vi "TempSetpointSetup.vi"(0 "Elevator Switch":bool=TRUE, 2 "Enable Auto":bool=TRUE, 3 "Elevator Manual Power":dbl format="%#_13g", 4 "Wrist Manual Power":dbl format="%#_13g", 5 "Horse Drive Manual Power":dbl format="%#_13g", 6 "Elevator Level Select":T1(ring), 7 "Wrist":T4(ring), 8 "Cluster":T2={"Elevator Setpoints"=[], "Wrist Setpoints"=[], "Horse Drive Setpoints"=[], "Wrist Gains"={"proportional gain (Kc)"=1.0, "integral time (Ti, min)"=0.01, "derivative time (Td, min)"=0.0}, "Wrist Power Limits"={"output high"=0.25, "output low"=-0.25}, "Horse Gains"={"proportional gain (Kc)"=1.0, "integral time (Ti, min)"=0.01, "derivative time (Td, min)"=0.0}, "Horse Power Limits"={"output high"=0.25, "output low"=-0.25}, "Elevator Gains"={"proportional gain (Kc)"=1.0, "integral time (Ti, min)"=0.01, "derivative time (Td, min)"=0.0}, "Elevator Power Limits"={"output high"=0.25, "output low"=-0.25}}, 9 "Horse Drive":T3(ring)) -> (20 "Elevator Power Out":dbl, 21 "Wrist Power Out":dbl, 22 "Horse Drive Power Out":dbl)   [LabVIEW 2018]
uses:
  <vilib>/Rock Robotics/WPI/ThirdParty/Phoenix-LabVIEW/Motor Controller/Get/CTRE_Phoenix_MotorController_GetSelectedSensorData.vi
  Toolbox/Simple Limit Switch/Limits(SingleSwitch).vi
  Toolbox/Simple Limit Switch/Limits(DoubleSwitch).vi
  Toolbox/Simple Limit Switch/Limits(Switch+Encoder).vi
panel:
  out "Outer Lift Limit":i32
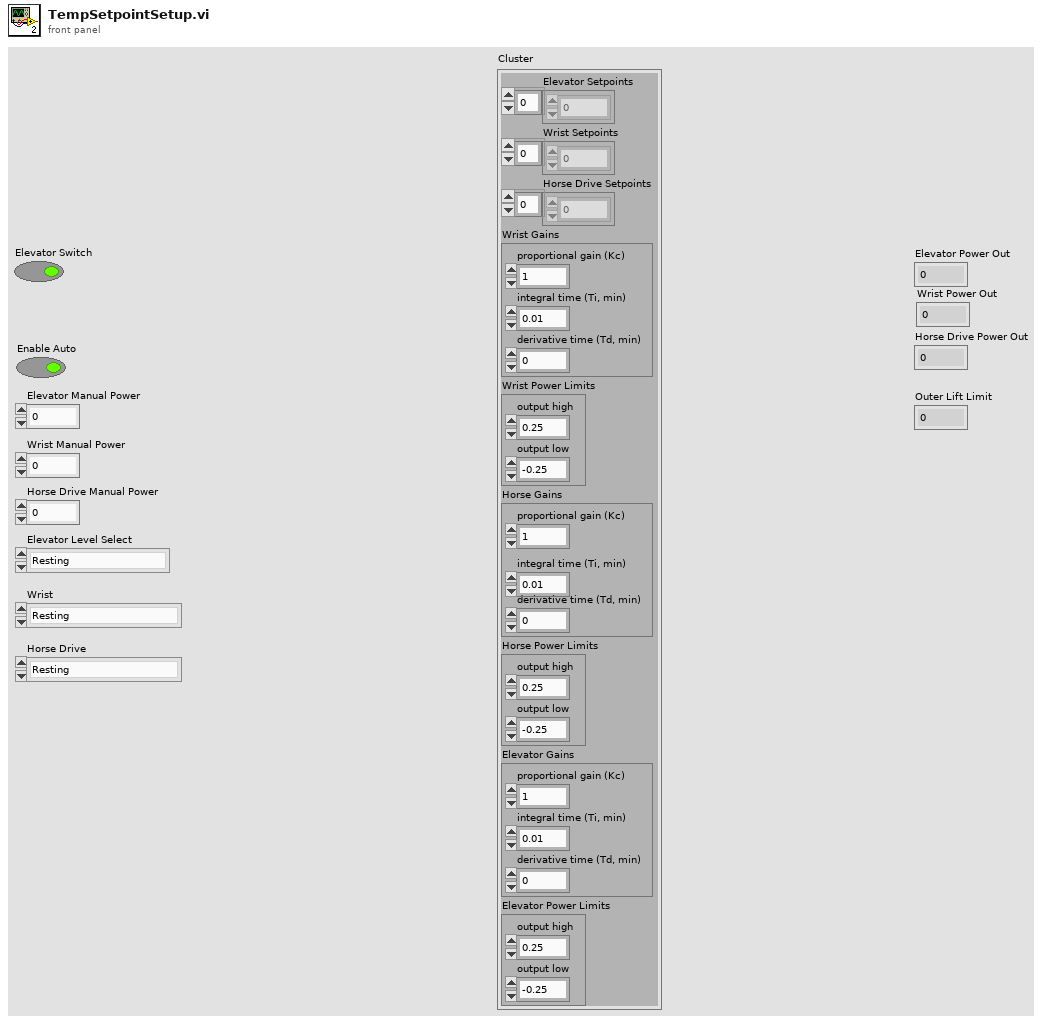
[diagram p1: front panel]
types:
  T1 = enum16{"Resting", "CargoShip Front", "CargoShip Back", "Cargo Mid", "Hatch Mid", "All High", "Cargo Intake"}
  T2 = cluster{"Elevator Setpoints":dbl[], "Wrist Setpoints":dbl[], "Horse Drive Setpoints":dbl[], "Wrist Gains":cluster{"proportional gain (Kc)":dbl, "integral time (Ti, min)":dbl, "derivative time (Td, min)":dbl}, "Wrist Power Limits":cluster{"output high":dbl, "output low":dbl}, "Horse Gains":cluster{"proportional gain (Kc)":dbl, "integral time (Ti, min)":dbl, "derivative time (Td, min)":dbl}, "Horse Power Limits":cluster{"output high":dbl, "output low":dbl}, "Elevator Gains":cluster{"proportional gain (Kc)":dbl, "integral time (Ti, min)":dbl, "derivative time (Td, min)":dbl}, "Elevator Power Limits":cluster{"output high":dbl, "output low":dbl}}
  T3 = enum16{"Resting", "PLACEHOLDER", "Hatch Intake", "Lift"}
  T4 = enum16{"Resting", "Hatch Ground Intake", "Hatch Place Low/Mid/CargoShip", "Hatch Place High", "Cargo Ground Intake", "Cargo Place Low/Mid", "Cargo Place High", "CargoShip Place Front", "CargoShip Place Back"}
  T5 = cluster{"proportional gain (Kc)":dbl, "integral time (Ti, min)":dbl, "derivative time (Td, min)":dbl}
  T6 = typedef "WPI_SwitchDevRef.ctl" = cluster{"DevStatus":errorcluster, "DIO Channel":T7, "CntIndex":T8, "Normally Closed":bool}
  T7 = typedef "FPGA_DIOChannel.ctl" = enum8{"DIO 0", "DIO 1", "DIO 2", "DIO 3", "DIO 4", "DIO 5", "DIO 6", "DIO 7", "DIO 8", "DIO 9", "DIO MXP 0", "DIO MXP 1", "DIO MXP 2", "DIO MXP 3", "DIO MXP 4", "DIO MXP 5", "DIO MXP 6", "DIO MXP 7", "DIO MXP 8", "DIO MXP 9", "DIO MXP 10", "DIO MXP 11", "DIO MXP 12", "DIO MXP 13", "DIO MXP 14", "DIO MXP 15", "SPI Port CS1", "SPI Port CS2", "SPI Port CS3", "SPI Port MISO", "SPI Port MOSI", "Invalid"}
  T8 = typedef "FPGA_CounterCtrSystemIndex.ctl" = enum8{"Ctr 0", "Ctr 1", "Ctr 2", "Ctr 3", "Ctr 4", "Ctr 5", "Ctr 6", "Ctr 7", "Invalid"}
  T9 = typedef "WPI_MotorControlDeviceRef.ctl" = cluster{"DeviceStatus":errorcluster, "Type":T10, "PWM":cluster{"PWM Channel":T11, "DeadBand":T12}, "CAN":cluster{"Device Number":u8, "SetOutput VI Ref":variant, "GetOutput VI Ref":variant, "Enable VI Ref":variant, "Disable VI Ref":variant, "Data":variant}, "Invert":bool, "DIO PWM":cluster{"PWM \"Enable\" Channel":T11, "DIOChannel":T7, "PWM Rate":dbl}}
  T10 = typedef "WPI_MotorControlType.ctl" = enum16{"PWM", "CAN", "DIO PWM"}
  T11 = typedef "FPGA_DIOPWMChannel.ctl" = enum8{"PWM 0", "PWM 1", "PWM 2", "PWM 3", "PWM 4", "PWM 5", "PWM 6", "PWM 7", "PWM 8", "PWM 9", "PWM MXP 0", "PWM MXP 1", "PWM MXP 2", "PWM MXP 3", "PWM MXP 4", "PWM MXP 5", "PWM MXP 6", "PWM MXP 7", "PWM MXP 8", "PWM MXP 9", "Invalid"}
  T12 = typedef "WPI_PWMDeadband.ctl" = cluster{"Name":string, "maxPositivePwm":i32, "minPositivePwm":i32, "centerPwm":i32, "maxNegativePwm":i32, "minNegativePwm":i32, "angularRange":u16}
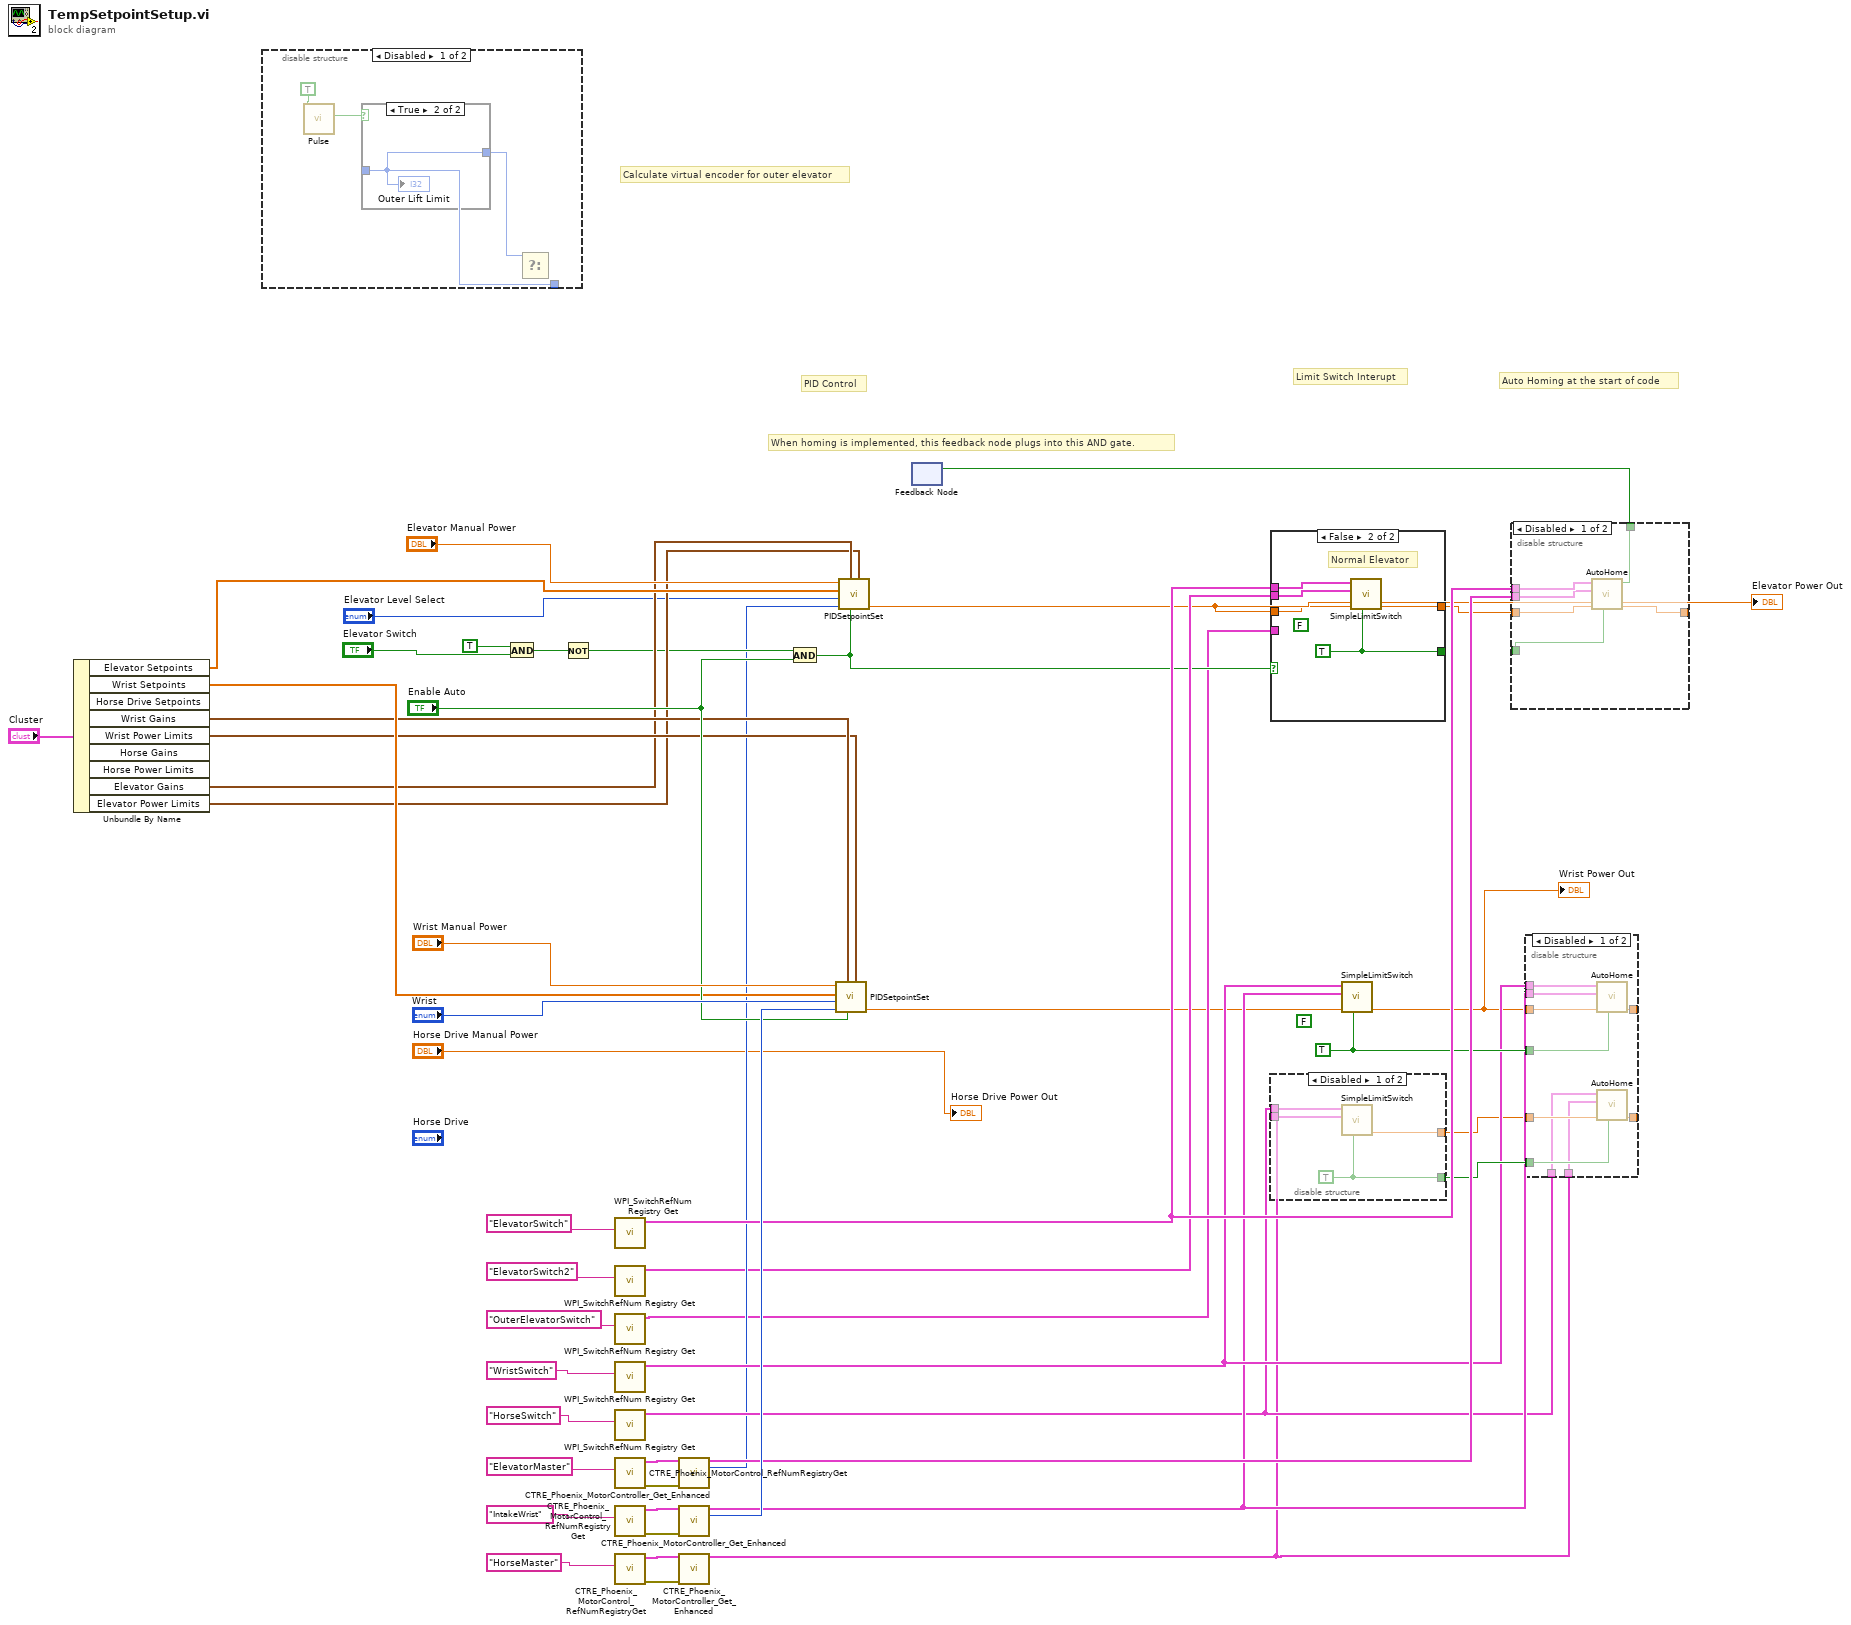
[diagram p0: block diagram]
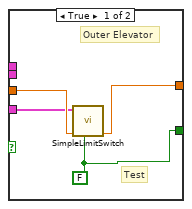
[diagram p3: hidden frame]
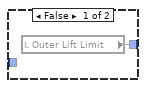
[diagram p4: hidden frame]
diagram:
  w35 = TRUE ("Into Limit Is Pos")
  (unwired) FALSE ("Into Limit Is Pos")
  # "When homing is implemented, this feedback node plugs into this AND gate."
  # "Calculate virtual encoder for outer elevator"
  # "Auto Homing at the start of code"
  # "Limit Switch Interupt"
  # "PID Control"
  n1 = Unbundle By Name("Cluster") -> ("Elevator Setpoints"=w25:dbl[], "Wrist Setpoints"=w24:dbl[], "Wrist Gains"=w23:T5, "Wrist Power Limits"=w22:cluster{"output high":dbl, "output low":dbl}, "Elevator Gains"=w21:T5, "Elevator Power Limits"=w20:cluster{"output high":dbl, "output low":dbl})  [unwired: 3 out]
  n2 = disable-structure shown="Disabled" {
    disable-tunnel: _ -> [w51 _]
    frame Disabled {
      n3 = call "Pulse.vi"("Rising Edge?"=TRUE) -> ("Output"=w53:bool)  [unwired: 10 in]
      n4 = case shown="True" w53 {
        tunnel: w51 -> [_ w56]
        tunnel: [w55 w56] -> w52
        frame False {
          n5 = local read "Outer Lift Limit"() -> (w55:i32)
        }
        frame True {
          "Outer Lift Limit" <- w56
        }
      }
      n6 = Select(t=w52) -> ()  [unwired: 2 in, 1 out]
    }
    frame Enabled {
    }
  }
  n7 = And(x=TRUE, y="Elevator Switch") -> (x .and. y?=w10:bool)
  n8 = Not(x=w10) -> (.not. x?=w18:bool)
  n9 = call <vilib>:"WPI_SwitchRefNum Registry Get.vi"("refnum name"="ElevatorSwitch") -> ("SwitchDevRef"=w37:T6)  [unwired: 9 in, 1 out]
  n10 = call <vilib>:"WPI_SwitchRefNum Registry Get.vi"("refnum name"="ElevatorSwitch2") -> ("SwitchDevRef"=w12:T6)  [unwired: 9 in, 1 out]
  n11 = call <vilib>:"WPI_SwitchRefNum Registry Get.vi"("refnum name"="OuterElevatorSwitch") -> ("SwitchDevRef"=w4:T6)  [unwired: 9 in, 1 out]
  n12 = call <vilib>:"WPI_SwitchRefNum Registry Get.vi"("refnum name"="WristSwitch") -> ("SwitchDevRef"=w33:T6)  [unwired: 9 in, 1 out]
  n13 = call <vilib>:"WPI_SwitchRefNum Registry Get.vi"("refnum name"="HorseSwitch") -> ("SwitchDevRef"=w31:T6)  [unwired: 9 in, 1 out]
  n14 = call <vilib>:"CTRE_Phoenix_MotorControl_RefNumRegistryGet.vi"("refnum name"="ElevatorMaster") -> ("error out"=w43:errorcluster, "PhoenixMotorControlDevRef"=w44:T9)  [unwired: 9 in]
  n15 = call <vilib>:"CTRE_Phoenix_MotorControl_RefNumRegistryGet.vi"("refnum name"="IntakeWrist") -> ("error out"=w41:errorcluster, "PhoenixMotorControlDevRef"=w42:T9)  [unwired: 9 in]
  n16 = call <vilib>:"CTRE_Phoenix_MotorControl_RefNumRegistryGet.vi"("refnum name"="HorseMaster") -> ("error out"=w39:errorcluster, "PhoenixMotorControlDevRef"=w40:T9)  [unwired: 9 in]
  n17 = call-poly <vilib>:"CTRE_Phoenix_MotorController_Get_Enhanced.vi"("PhoenixMotorControlDevRef"=w44, "error in"=w43) -> ("PhoenixMotorControlDevRef"=w36:T9, "Position (Raw Sensor Units)"=w17:i32)  [unwired: 10 in, 2 out]
  n18 = call-poly <vilib>:"CTRE_Phoenix_MotorController_Get_Enhanced.vi"("PhoenixMotorControlDevRef"=w42, "error in"=w41) -> ("PhoenixMotorControlDevRef"=w32:T9, "Position (Raw Sensor Units)"=w38:i32)  [unwired: 10 in, 2 out]
  n19 = call-poly <vilib>:"CTRE_Phoenix_MotorController_Get_Enhanced.vi"("PhoenixMotorControlDevRef"=w40, "error in"=w39) -> ("PhoenixMotorControlDevRef"=w30:T9)  [unwired: 10 in, 3 out]
  n20 = And(x=w18, y="Enable Auto") -> (x .and. y?=w7:bool)
  n21 = call "PIDSetpointSet.vi"("Output Range"=w22, "Auto"="Enable Auto", "PID Gains"=w23, "Encoder Position"=w38, "Level"="Wrist", "Setpoints"=w24, "Manual Power"="Wrist Manual Power") -> ("Power Out"=w2:dbl)  [unwired: 4 in]
  n22 = call "PIDSetpointSet.vi"("Output Range"=w20, "Auto"=w7, "PID Gains"=w21, "Encoder Position"=w17, "Level"="Elevator Level Select", "Setpoints"=w25, "Manual Power"="Elevator Manual Power") -> ("Power Out"=w5:dbl)  [unwired: 4 in]
  "Elevator Power Out" <- w5
  n23 = feedback #1() -> ()  [unwired: 2 in]
  n24 = case shown="False" w7 {
    tunnel: w5 -> [w59 w65]
    tunnel: w37 -> [_ w64]
    tunnel: w12 -> [_ w63]
    tunnel: [w57 w62] -> _
    tunnel: [w60 w61] -> w27
    tunnel: w4 -> [w58 _]
    frame True {
      w57 = FALSE ("Into Home Limit Is Pos")
      # "Test"
      # "Outer Elevator"
      n25 = call-poly "SimpleLimitSwitch.vi"("Into Home Limit Is Pos (Motor)"=w57, "Power In"=w59, "Limit Switch Ref"=w58) -> ("Power Out"=w60:dbl)  [unwired: 8 in]
    }
    frame False {
      w62 = TRUE ("Into Limit Is Pos")
      (unwired) FALSE ("Into Limit Is Pos")
      # "Normal Elevator"
      n26 = call-poly "SimpleLimitSwitch.vi"("Into Home Limit Is Pos"=w62, "Power In"=w65, "2nd Limit Switch Ref"=w63, "Home Limit Switch Ref"=w64) -> ("Power Out"=w61:dbl)  [unwired: 7 in]
    }
  }
  n27 = disable-structure shown="Disabled" {
    disable-tunnel: [w69 _] -> w34
    disable-tunnel: w31 -> [w68 _]
    disable-tunnel: w30 -> [w67 _]
    disable-tunnel: [w66 _] -> w28
    frame Disabled {
      w69 = TRUE ("Into Limit Is Pos")
      n28 = call-poly "SimpleLimitSwitch.vi"("Into Home Limit Is Pos (Motor)"=w69, "Motor Ref"=w67, "Limit Switch Ref"=w68) -> ("Power Out"=w66:dbl)  [unwired: 8 in]
    }
    frame Enabled {
    }
  }
  n29 = call-poly "SimpleLimitSwitch.vi"("Into Home Limit Is Pos (Motor)"=w35, "Power In"=w2, "Motor Ref"=w32, "Limit Switch Ref"=w33) -> ("Power Out"=w3:dbl)  [unwired: 7 in]
  "Wrist Power Out" <- w3
  n30 = disable-structure shown="Disabled" {
    disable-tunnel: w27 -> [w75 _]
    disable-tunnel: [w74 _] -> _
    disable-tunnel: w37 -> [w73 _]
    disable-tunnel: w36 -> [w72 _]
    disable-tunnel: _ -> [w71 _]
    disable-tunnel: [w70 _] -> w9
    frame Disabled {
      n31 = call "AutoHome.vi"("Into Home Limit Is Pos"=w71, "Power In"=w75, "Motor Ref"=w72, "Limit Switch Ref"=w73) -> ("Power Out"=w74:dbl, "Done"=w70:bool)  [unwired: 6 in]
    }
    frame Enabled {
    }
  }
  n32 = feedback-in #1(w9) -> ()
  n33 = disable-structure shown="Disabled" {
    disable-tunnel: w3 -> [w85 _]
    disable-tunnel: [w84 _] -> _
    disable-tunnel: w28 -> [w83 _]
    disable-tunnel: [w82 _] -> _
    disable-tunnel: w35 -> [w81 _]
    disable-tunnel: w34 -> [w80 _]
    disable-tunnel: w33 -> [w79 _]
    disable-tunnel: w32 -> [w78 _]
    disable-tunnel: w31 -> [w77 _]
    disable-tunnel: w30 -> [w76 _]
    frame Disabled {
      n34 = call "AutoHome.vi"("Into Home Limit Is Pos"=w81, "Power In"=w85, "Motor Ref"=w78, "Limit Switch Ref"=w79) -> ("Power Out"=w84:dbl)  [unwired: 6 in, 1 out]
      n35 = call "AutoHome.vi"("Into Home Limit Is Pos"=w80, "Power In"=w83, "Motor Ref"=w76, "Limit Switch Ref"=w77) -> ("Power Out"=w82:dbl)  [unwired: 6 in, 1 out]
    }
    frame Enabled {
    }
  }
  "Horse Drive Power Out" <- "Horse Drive Manual Power"
